vi "TDMS_Slicer.vi"() -> ()   [LabVIEW 2016]
doc: "TDMS로 저장된 파일을 읽고 추출함"
uses:
  Control/control_state.ctl
  <vilib>/Utility/error.llb/DialogType.ctl
panel:
  in  "Tach CH":i32=1
  out "RPM":dbl
  in  "Set input":i32
  in  "CH input":i32
  out "Measured time":string
  out "Error Out":errorcluster caption="에러 출력"
  in  "Error In":errorcluster caption="에러 입력"
  out "Channel number":string
  in  "Provious Set":bool
  in  "Next Set":bool
  in  "Provious CH":bool
  out "Data set number":string
  in  "Save name":string="FileNAME"
  out "TDMS Path":path
  out "Graph":waveform(dbl)(graph)
  out "TDMS_info":T1
  in  "END":bool
  in  "SAVE":bool
  in  "Next CH":bool
  in  "OPEN":bool
  # "TDMS read and extraction program by Kyuman Kim"
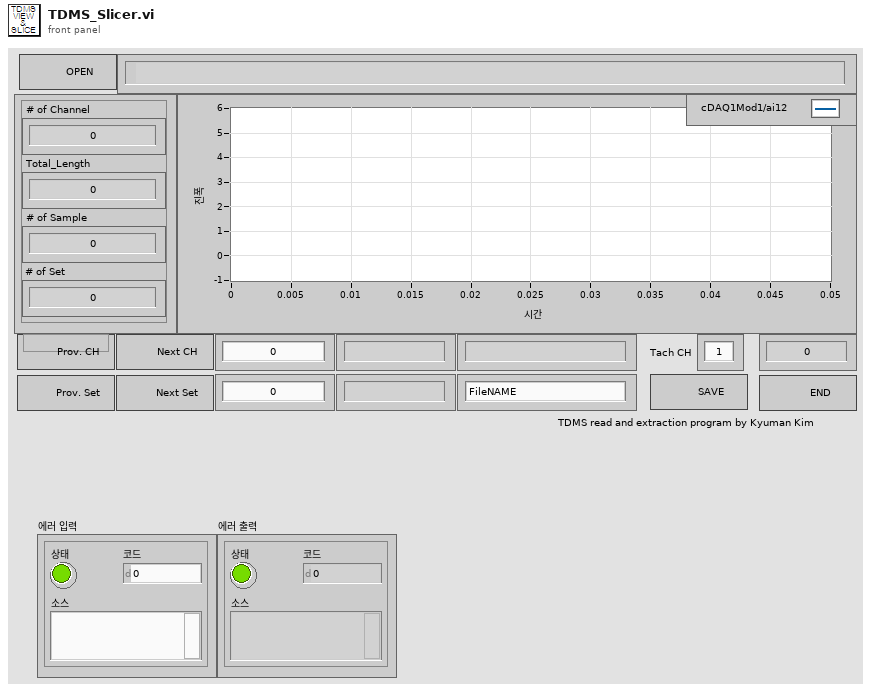
[diagram p1: front panel]
types:
  T1 = cluster{"# of Channel":i32, "Total_Length":u64, "# of Sample":i32, "# of Set":i32}
  T2 = typedef "control_state.ctl" = enum16{"Init", "Wait", "Setup", "Open", "Read", "Save", "End", "Error"}
  T3 = cluster{"# of Channel":i32, "Total_Length":u64, "# of Sample":i32, "# of Set":dbl}
  T4 = typedef "DialogType.ctl" = u16
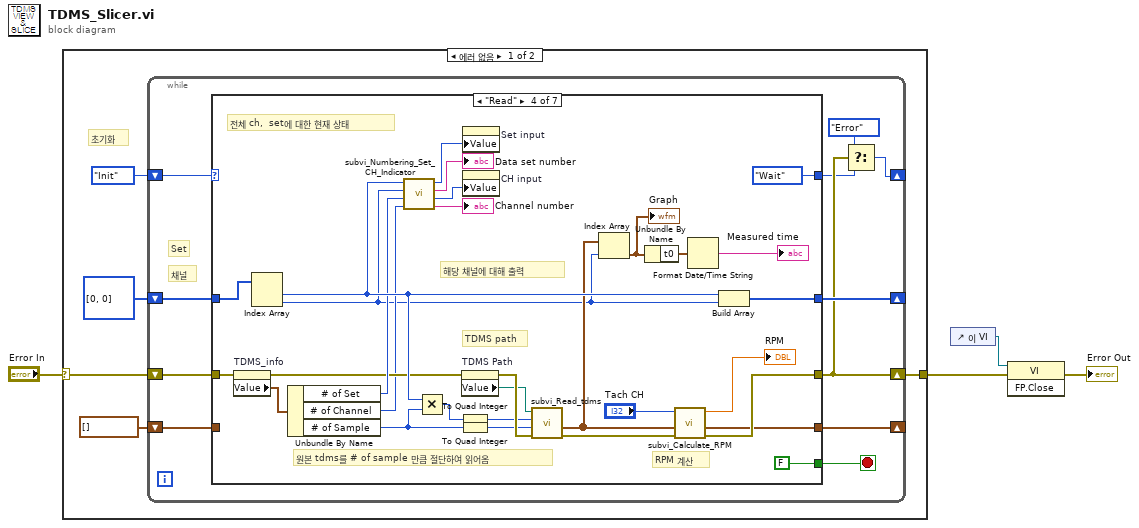
[diagram p0: block diagram]
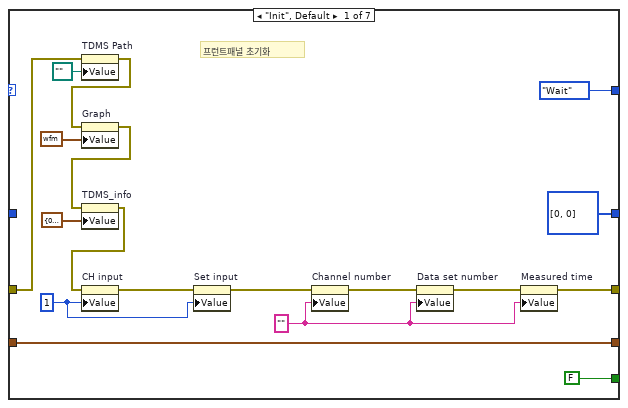
[diagram p2: hidden frame]
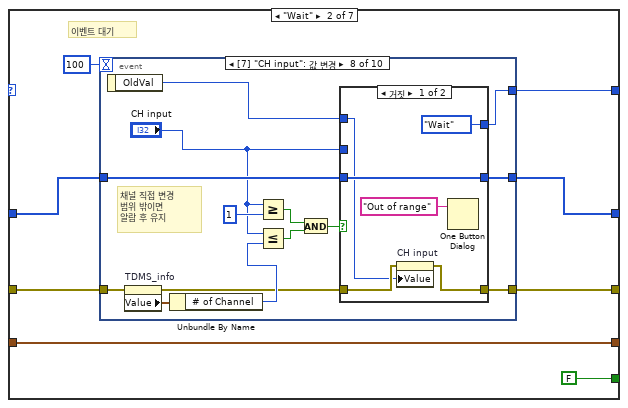
[diagram p3: hidden frame]
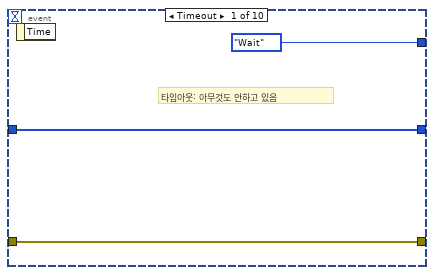
[diagram p4: hidden frame]
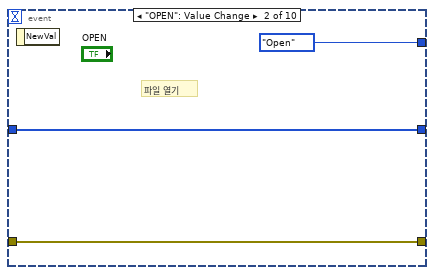
[diagram p5: hidden frame]
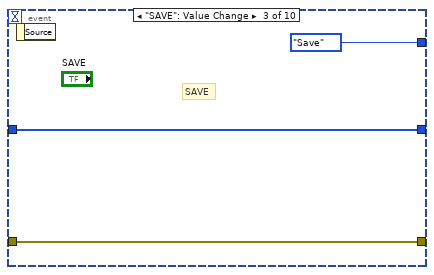
[diagram p6: hidden frame]
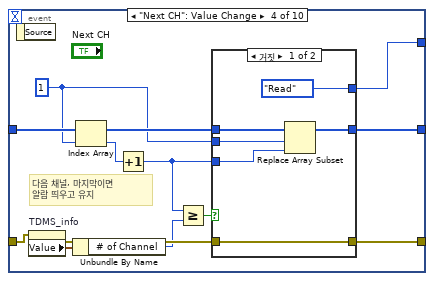
[diagram p7: hidden frame]
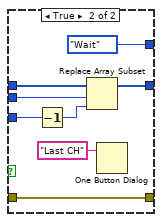
[diagram p8: hidden frame]
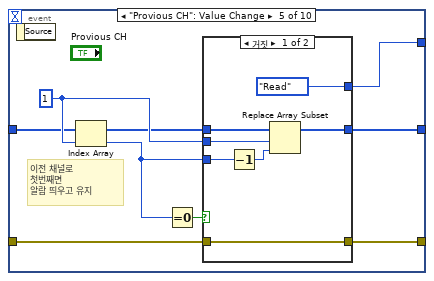
[diagram p9: hidden frame]
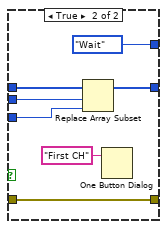
[diagram p10: hidden frame]
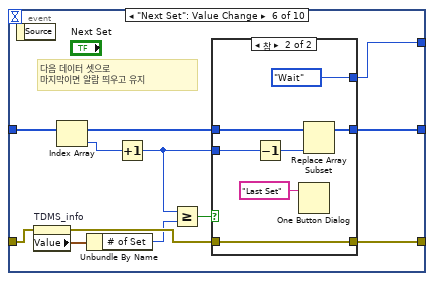
[diagram p11: hidden frame]
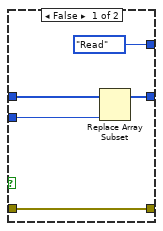
[diagram p12: hidden frame]
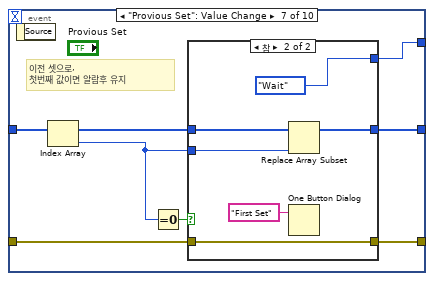
[diagram p13: hidden frame]
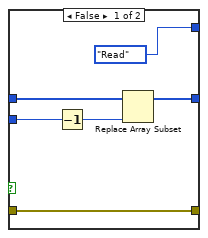
[diagram p14: hidden frame]
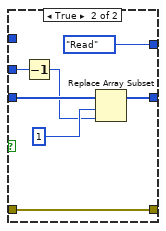
[diagram p15: hidden frame]
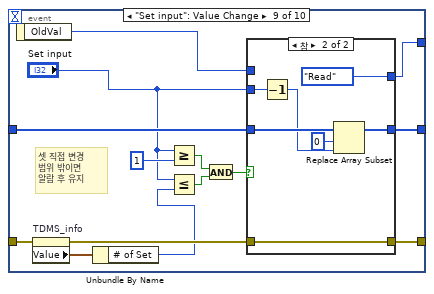
[diagram p16: hidden frame]
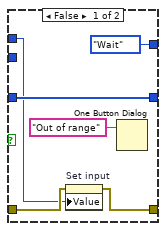
[diagram p17: hidden frame]
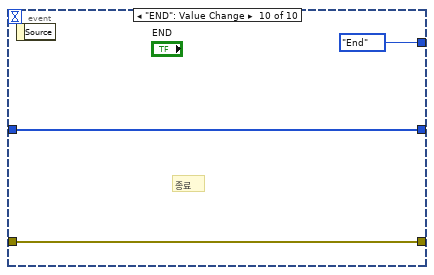
[diagram p18: hidden frame]
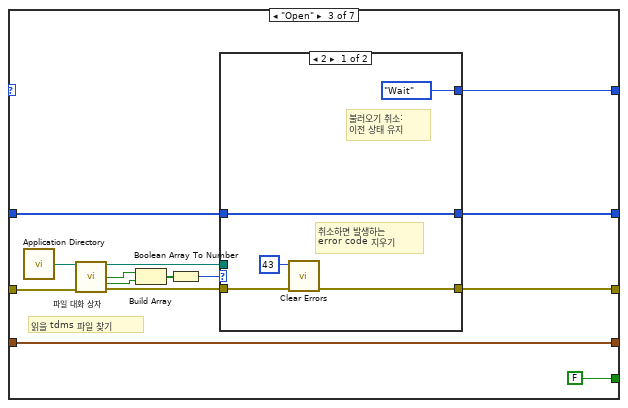
[diagram p19: hidden frame]
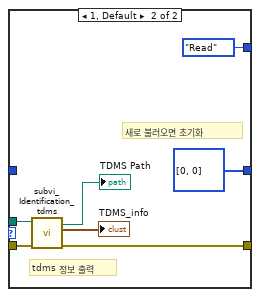
[diagram p20: hidden frame]
diagram:
  n1 = case shown="에러 없음" "Error In" {
    selector: "Error In" -> [w6 w309]
    tunnel: [w5 w309] -> w2
    frame No Error {
      # "초기화"
      n2 = while {
        shift-right: [w18] -> _
        shift-left: waveform(dbl)[] [] ("data") -> [w17]
        shift-right: [w16] -> _
        shift-left: i32[] [0, 0] -> [w19]
        shift-right: [w12] -> _
        shift-left: control_state."Init" ("열거형") -> [w20]
        shift-right: [w11] -> w5
        shift-left: w6 -> [w15]
        stop <- w14 stop-if-true
        # "채널"
        # "Set"
        n3 = case shown="\"Read\"" w20 {
          tunnel: w19 -> [_ w41 w205 w250 w265 _ _]
          tunnel: [FALSE FALSE FALSE FALSE FALSE w271 TRUE] -> w14
          tunnel: [w33 w43 w212 w231 w262 w277 waveform(dbl)[] [] ("data")] -> w18
          tunnel: w17 -> [w33 w43 w212 _ w262 w277 _]
          tunnel: [i32[] [0, 0] w42 w206 w248 w265 i32[] [] i32[] []] -> w16
          tunnel: [control_state."Wait" ("열거형") w44 w203 control_state."Wait" ("열거형") control_state."Wait" ("열거형") w274 control_state."Init" ("열거형")] -> w10
          tunnel: w15 -> [w38 w39 w211 w245 w267 w273 w303]
          tunnel: [w29 w40 w204 w234 w258 w272 w301] -> w11
          frame "Init", Default {
            w22 = 1 ("CH input")
            w23 = "" ("Channel number")
            # "프런트패널 초기화"
            n4 = property on="TDMS Path" class="Path"(error in=w38, "Value"=path "" ("TDMS Path")) -> (error out=w25:errorcluster)  [unwired: 1 in, 1 out]
            n5 = property on="Graph" class="WFGraph (엄격한)"(error in=w25, "Value"=waveform(dbl) {"t0"=timestamp(3735946803.3210297 s since 1904-01-01), "dt"=4.8824999999999954e-05, "Y"=[], "attributes"=variant("NI_ChannelName"=variant(string "cDAQ1Mod1/ai12"), "NI_UnitDescription"=variant(string "Volts"))} ("Graph")) -> (error out=w37:errorcluster)  [unwired: 1 in, 1 out]
            n6 = property on="TDMS_info" class="Clust (엄격한)"(error in=w37, "Value"=T3 {"# of Channel"=0, "Total_Length"=0, "# of Sample"=0, "# of Set"=0.0} ("TDMS_info")) -> (error out=w36:errorcluster)  [unwired: 1 in, 1 out]
            n7 = property on="CH input" class="DigNum (엄격한)"(error in=w36, "Value"=w22) -> (error out=w27:errorcluster)  [unwired: 1 in, 1 out]
            n8 = property on="Set input" class="DigNum (엄격한)"(error in=w27, "Value"=w22) -> (error out=w26:errorcluster)  [unwired: 1 in, 1 out]
            n9 = property on="Channel number" class="Str"(error in=w26, "Value"=w23) -> (error out=w30:errorcluster)  [unwired: 1 in, 1 out]
            n10 = property on="Data set number" class="Str"(error in=w30, "Value"=w23) -> (error out=w28:errorcluster)  [unwired: 1 in, 1 out]
            n11 = property on="Measured time" class="Str"(error in=w28, "Value"=w23) -> (error out=w29:errorcluster)  [unwired: 1 in, 1 out]
          }
          frame "Wait" {
            # "이벤트 대기"
            n12 = event shown="[7] \"CH input\": 값 변경" {
              selector: _ -> [_ _ _ _ _ _ _ _ _ _]
              dyn-events: _ -> [_ _ _ _ _ _ _ _ _ _]
              timeout: 100 -> [_ _ _ _ _ _ _ _ _ _]
              tunnel: [control_state."Wait" ("열거형") control_state."Open" ("열거형") control_state."Save" ("열거형") w62 w85 w106 w130 w159 w175 control_state."End" ("열거형")] -> w44
              tunnel: w41 -> [w48 w51 w54 w66 w88 w112 w133 w158 w178 w201]
              tunnel: [w48 w51 w54 w63 w87 w111 w132 w157 w176 w201] -> w42
              tunnel: [w47 w50 w53 w56 w82 w104 w128 w153 w183 w200] -> w40
              tunnel: w39 -> [w47 w50 w53 w57 w83 w105 w127 w154 w182 w200]
              event Timeout {
                # "타임아웃: 아무것도 안하고 있음"
                n13 = event-data() -> ()  [unwired: 1 in, 1 out]
              }
              event "OPEN": Value Change {
                # "파일 열기"
                n14 = event-data() -> ()  [unwired: 1 in, 1 out]
              }
              event "SAVE": Value Change {
                # "SAVE"
                n15 = event-data() -> ()  [unwired: 1 in, 1 out]
              }
              event "Next CH": Value Change {
                w64 = 1 ("인덱스")
                # "다음 채널, 마지막이면\n알람 띄우고 유지"
                n16 = event-data() -> ()  [unwired: 1 in, 1 out]
                n17 = property on="TDMS_info" class="Clust (엄격한)"(error in=w57) -> (error out=w67:errorcluster, "Value"=w61:T1)  [unwired: 1 in, 1 out]
                n18 = Unbundle By Name(w61) -> ("# of Channel"=w60:i32)
                n19 = Index Array(array=w66, index=w64) -> (element=w65:i32)
                n20 = Increment(x=w65) -> (x+1=w58:i32)
                n21 = Greater Or Equal?(x=w58, y=w60) -> (x >= y?=w59:bool)
                n22 = case shown="거짓" w59 {
                  tunnel: w66 -> [w72 w81]
                  tunnel: w58 -> [w70 w80]
                  tunnel: w64 -> [w71 w79]
                  tunnel: [w73 w78] -> w63
                  tunnel: [control_state."Read" ("열거형") control_state."Wait" ("열거형")] -> w62
                  tunnel: w67 -> [w68 w74]
                  tunnel: [w68 w74] -> w56
                  frame False {
                    n23 = Replace Array Subset(array=w72, new element=w70, index=w71) -> (w73:i32[])
                  }
                  frame True {
                    n24 = Decrement(x=w80) -> (x-1=w76:i32)
                    n25 = Replace Array Subset(array=w81, new element=w76, index=w79) -> (w78:i32[])
                    n26 = One Button Dialog(message="Last CH" ("메시지")) -> ()  [unwired: 1 in, 1 out]
                  }
                }
              }
              event "Provious CH": Value Change {
                w89 = 1 ("인덱스")
                # "이전 채널로\n첫번째면\n알람 띄우고 유지"
                n27 = event-data() -> ()  [unwired: 1 in, 1 out]
                n28 = Index Array(array=w88, index=w89) -> (element=w84:i32)
                n29 = Equal To 0?(x=w84) -> (x = 0?=w86:bool)
                n30 = case shown="거짓" w86 {
                  tunnel: w84 -> [w95 w98]
                  tunnel: w89 -> [w96 w103]
                  tunnel: w88 -> [w93 w102]
                  tunnel: [w94 w101] -> w87
                  tunnel: [control_state."Read" ("열거형") control_state."Wait" ("열거형")] -> w85
                  tunnel: w83 -> [w90 w97]
                  tunnel: [w90 w97] -> w82
                  frame False {
                    n31 = Decrement(x=w95) -> (x-1=w91:i32)
                    n32 = Replace Array Subset(array=w93, new element=w91, index=w96) -> (w94:i32[])
                  }
                  frame True {
                    n33 = Replace Array Subset(array=w102, new element=w98, index=w103) -> (w101:i32[])
                    n34 = One Button Dialog(message="First CH" ("메시지")) -> ()  [unwired: 1 in, 1 out]
                  }
                }
              }
              event "Next Set": Value Change {
                # "다음 데이터 셋으로\n마지막이면 알람 띄우고 유지"
                n35 = event-data() -> ()  [unwired: 1 in, 1 out]
                n36 = property on="TDMS_info" class="Clust (엄격한)"(error in=w105) -> (error out=w114:errorcluster, "Value"=w110:T1)  [unwired: 1 in, 1 out]
                n37 = Index Array(array=w112) -> (element=w113:i32)  [unwired: 1 in]
                n38 = Unbundle By Name(w110) -> ("# of Set"=w108:i32)
                n39 = Increment(x=w113) -> (x+1=w107:i32)
                n40 = Greater Or Equal?(x=w107, y=w108) -> (x >= y?=w109:bool)
                n41 = case shown="참" w109 {
                  tunnel: w107 -> [w117 w126]
                  tunnel: w112 -> [w119 w125]
                  tunnel: [w118 w124] -> w111
                  tunnel: [control_state."Read" ("열거형") control_state."Wait" ("열거형")] -> w106
                  tunnel: [w115 w120] -> w104
                  tunnel: w114 -> [w115 w120]
                  frame False {
                    n42 = Replace Array Subset(array=w119, new element=w117) -> (w118:i32[])  [unwired: 1 in]
                  }
                  frame True {
                    n43 = Decrement(x=w126) -> (x-1=w123:i32)
                    n44 = One Button Dialog(message="Last Set" ("메시지")) -> ()  [unwired: 1 in, 1 out]
                    n45 = Replace Array Subset(array=w125, new element=w123) -> (w124:i32[])  [unwired: 1 in]
                  }
                }
              }
              event "Provious Set": Value Change {
                # "이전 셋으로,\n첫번째 값이면 알람후 유지"
                n46 = event-data() -> ()  [unwired: 1 in, 1 out]
                n47 = Index Array(array=w133) -> (element=w129:i32)  [unwired: 1 in]
                n48 = Equal To 0?(x=w129) -> (x = 0?=w131:bool)
                n49 = case shown="참" w131 {
                  tunnel: w133 -> [w138 w145]
                  tunnel: [w137 w144] -> w132
                  tunnel: w129 -> [w139 w141]
                  tunnel: [control_state."Read" ("열거형") control_state."Wait" ("열거형")] -> w130
                  tunnel: [w134 w140] -> w128
                  tunnel: w127 -> [w134 w140]
                  frame False {
                    n50 = Decrement(x=w139) -> (x-1=w135:i32)
                    n51 = Replace Array Subset(array=w138, new element=w135) -> (w137:i32[])  [unwired: 1 in]
                  }
                  frame True {
                    n52 = Replace Array Subset(array=w145, new element=w141) -> (w144:i32[])  [unwired: 1 in]
                    n53 = One Button Dialog(message="First Set" ("메시지")) -> ()  [unwired: 1 in, 1 out]
                  }
                }
              }
              event "CH input": Value Change {
                # "채널 직접 변경\n범위 밖이면\n알람 후 유지"
                n54 = event-data() -> ("OldVal"=w148:i32)  [unwired: 1 in]
                n55 = property on="TDMS_info" class="Clust (엄격한)"(error in=w154) -> (error out=w147:errorcluster, "Value"=w156:T1)  [unwired: 1 in, 1 out]
                n56 = Unbundle By Name(w156) -> ("# of Channel"=w149:i32)
                n57 = Greater Or Equal?(x="CH input", y=1) -> (x >= y?=w151:bool)
                n58 = Less Or Equal?(x="CH input", y=w149) -> (x <= y?=w150:bool)
                n59 = And(x=w151, y=w150) -> (x .and. y?=w152:bool)
                n60 = case shown="거짓" w152 {
                  tunnel: [control_state."Wait" ("열거형") control_state."Read" ("열거형")] -> w159
                  tunnel: w158 -> [w164 w171]
                  tunnel: [w164 w170] -> w157
                  tunnel: w147 -> [w162 w167]
                  tunnel: [w161 w167] -> w153
                  tunnel: "CH input" -> [_ w166]
                  tunnel: w148 -> [w160 _]
                  frame False {
                    n61 = property on="CH input" class="DigNum (엄격한)"(error in=w162, "Value"=w160) -> (error out=w161:errorcluster)  [unwired: 1 in, 1 out]
                    n62 = One Button Dialog(message="Out of range" ("메시지")) -> ()  [unwired: 1 in, 1 out]
                  }
                  frame True {
                    n63 = Decrement(x=w166) -> (x-1=w168:i32)
                    n64 = Replace Array Subset(array=w171, new element=w168, index=1 ("인덱스")) -> (w170:i32[])
                  }
                }
              }
              event "Set input": Value Change {
                # "셋 직접 변경\n범위 밖이면\n알람 후 유지"
                n65 = event-data() -> ("OldVal"=w177:i32)  [unwired: 1 in]
                n66 = property on="TDMS_info" class="Clust (엄격한)"(error in=w182) -> (error out=w181:errorcluster, "Value"=w180:T1)  [unwired: 1 in, 1 out]
                n67 = Unbundle By Name(w180) -> ("# of Set"=w179:i32)
                n68 = Greater Or Equal?(x="Set input", y=1) -> (x >= y?=w185:bool)
                n69 = Less Or Equal?(x="Set input", y=w179) -> (x <= y?=w184:bool)
                n70 = And(x=w185, y=w184) -> (x .and. y?=w174:bool)
                n71 = case shown="참" w174 {
                  tunnel: [control_state."Wait" ("열거형") control_state."Read" ("열거형")] -> w175
                  tunnel: w178 -> [w191 w198]
                  tunnel: [w191 w197] -> w176
                  tunnel: w181 -> [w189 w194]
                  tunnel: [w188 w194] -> w183
                  tunnel: w177 -> [w187 _]
                  tunnel: "Set input" -> [_ w193]
                  frame False {
                    n72 = property on="Set input" class="DigNum (엄격한)"(error in=w189, "Value"=w187) -> (error out=w188:errorcluster)  [unwired: 1 in, 1 out]
                    n73 = One Button Dialog(message="Out of range" ("메시지")) -> ()  [unwired: 1 in, 1 out]
                  }
                  frame True {
                    n74 = Decrement(x=w193) -> (x-1=w195:i32)
                    n75 = Replace Array Subset(array=w198, new element=w195, index=0 ("인덱스")) -> (w197:i32[])
                  }
                }
              }
              event "END": Value Change {
                # "종료"
                n76 = event-data() -> ()  [unwired: 1 in, 1 out]
              }
            }
          }
          frame "Open" {
            # "읽을 tdms 파일 찾기"
            n77 = call <vilib>:"Application Directory.vi"() -> ("Application Directory"=w216:path)
            n78 = call "파일 대화 상자"("start path"=w216, "error in"=w211) -> ("selected path"=w215:path, "exists"=w210:bool, "cancelled"=w209:bool, "error out"=w214:errorcluster)  [unwired: 10 in]
            n79 = Build Array(w210, w209) -> (w208:bool[])
            n80 = Boolean Array To Number(Boolean array=w208) -> (number=w207:u32)
            n81 = case shown="2" w207 {
              tunnel: w215 -> [_ w228]
              tunnel: w214 -> [w219 w227]
              tunnel: [control_state."Wait" ("열거형") control_state."Read" ("열거형")] -> w203
              tunnel: [w218 w225] -> w204
              tunnel: [w220 i32[] [0, 0]] -> w206
              tunnel: w205 -> [w220 _]
              frame 2 {
                # "취소하면 발생하는 \nerror code 지우기"
                # "불러오기 취소:\n이전 상태 유지"
                n82 = call <vilib>:"Clear Errors.vi"("error in (no error)"=w219, "specific error code to clear (0: all)"=43) -> ("error out"=w218:errorcluster)  [unwired: 4 in, 1 out]
              }
              frame 1, Default {
                # "새로 불러오면 초기화"
                # "tdms 정보 출력"
                n83 = call "subvi_Identification_tdms.vi"("Error In"=w227, "Path in"=w228) -> ("Error Out"=w225:errorcluster, "TDMS_info"=→"TDMS_info":T1, "Path out"=→"TDMS Path":path)  [unwired: 7 in]
              }
            }
          }
          frame "Read" {
            # "RPM 계산"
            # "TDMS path"
            # "해당 채널에 대해 출력"
            # "원본 tdms를 # of sample 만큼 절단하여 읽어옴"
            # "전체 ch,  set에 대한 현재 상태"
            n84 = property on="TDMS_info" class="Clust (엄격한)"(error in=w245) -> (error out=w240:errorcluster, "Value"=w256:T1)  [unwired: 1 in, 1 out]
            n85 = Index Array(array=w250) -> (element #1=w249:i32, element #2=w229:i32)  [unwired: 2 in]
            n86 = Unbundle By Name(w256) -> ("# of Set"=w241:i32, "# of Channel"=w235:i32, "# of Sample"=w253:i32)
            n87 = call "subvi_Numbering_Set_CH_Indicator.vi"("# of Channel"=w235, "# of Set"=w241, "CH data"=w229, "Set data"=w249) -> ("CH state"=→"Channel number":string, "CH value"=w237:i32, "Set state"=→"Data set number":string, "Set value"=w238:i32)  [unwired: 4 in]
            n88 = Multiply(x=w249, y=w253) -> (x*y=w252:i32)
            n89 = To Quad Integer(1:w252) -> (0:w254:i64)
            n90 = To Quad Integer(1:w253) -> (0:w255:i64)
            n91 = property on="TDMS Path" class="Path"(error in=w240) -> (error out=w257:errorcluster, "Value"=w239:path)  [unwired: 1 in, 1 out]
            n92 = property on="Set input" class="DigNum (엄격한)"("Value"=w238) -> ()  [unwired: 2 in, 2 out]
            n93 = property on="CH input" class="DigNum (엄격한)"("Value"=w237) -> ()  [unwired: 2 in, 2 out]
            n94 = call "subvi_Read_tdms.vi"("Error In"=w257, "카운트(-1: 전체)"=w255, "오프셋(0)"=w254, "selected path"=w239) -> ("Error Out"=w233:errorcluster, "data"=w231:waveform(dbl)[])  [unwired: 6 in]
            n95 = Index Array(array=w231, index=w229) -> (element=w244:waveform(dbl))
            "Graph" <- w244
            n96 = Unbundle By Name(w244) -> ("t0"=w243:timestamp)
            n97 = call "subvi_Calculate_RPM.vi"("에러 입력"=w233, "data"=w231, "Tach CH"="Tach CH") -> ("에러 출력"=w234:errorcluster, "RPM"=→"RPM":dbl)  [unwired: 7 in]
            n98 = Format Date/Time String(seconds (now)=w243) -> (date/time string=→"Measured time":string)  [unwired: 2 in]
            n99 = Build Array(w249, w229) -> (w248:i32[])
          }
          frame "Save" {
            # "어플리케이션 경로"
            # "그룹이름"
            # "어플리케이션 경로 밑에 TDMS_Sliced 폴더에 날짜_이름으로 저장"
            n100 = call <vilib>:"Application Directory.vi"() -> ("Application Directory"=w260:path)
            n101 = call "subvi_Save_tdms.vi"("data"=w262, "그룹 이름"="Sliced data" ("그룹 이름 입력(제목없음)"), "Error In"=w267, "Save name"="Save name", "appended path"=w260) -> ("Error Out"=w259:errorcluster)  [unwired: 6 in]
            n102 = flat-sequence {
              tunnel: [w268] -> w258
              tunnel: w259 -> [w268]
              frame #0 {
                n103 = One Button Dialog(message="Sliced TDMS\nSAVED" ("메시지")) -> ()  [unwired: 1 in, 1 out]
              }
            }
          }
          frame "End" {
            n104 = Two Button Dialog(message="끝냅니다" ("메시지")) -> (T button?=w275:bool)  [unwired: 2 in]
            n105 = case shown="거짓" w275 {
              tunnel: w273 -> [w280 w285]
              tunnel: [control_state."Wait" ("열거형") control_state."Init" ("열거형")] -> w274
              tunnel: [w280 w289] -> w272
              tunnel: [FALSE TRUE] -> w271
              frame False {
                # "아무것도 하지 않고 wait 이동"
              }
              frame True {
                w283 = "" ("Channel number")
                # "종료 전 초기화"
                n106 = property on="TDMS Path" class="Path"(error in=w285, "Value"=path "" ("TDMS Path")) -> (error out=w284:errorcluster)  [unwired: 1 in, 1 out]
                n107 = property on="Graph" class="WFGraph (엄격한)"(error in=w284, "Value"=waveform(dbl) {"t0"=timestamp(3735946803.3210297 s since 1904-01-01), "dt"=4.8824999999999954e-05, "Y"=[], "attributes"=variant("NI_ChannelName"=variant(string "cDAQ1Mod1/ai12"), "NI_UnitDescription"=variant(string "Volts"))} ("Graph")) -> (error out=w293:errorcluster)  [unwired: 1 in, 1 out]
                n108 = property on="TDMS_info" class="Clust (엄격한)"(error in=w293, "Value"=T3 {"# of Channel"=0, "Total_Length"=0, "# of Sample"=0, "# of Set"=0.0} ("TDMS_info")) -> (error out=w292:errorcluster)  [unwired: 1 in, 1 out]
                n109 = property on="CH input" class="DigNum (엄격한)"(error in=w292, "Value"=1 ("CH input")) -> (error out=w288:errorcluster)  [unwired: 1 in, 1 out]
                n110 = property on="Set input" class="DigNum (엄격한)"(error in=w288, "Value"=1 ("Set input")) -> (error out=w287:errorcluster)  [unwired: 1 in, 1 out]
                n111 = property on="Channel number" class="Str"(error in=w287, "Value"=w283) -> (error out=w291:errorcluster)  [unwired: 1 in, 1 out]
                n112 = property on="Data set number" class="Str"(error in=w291, "Value"=w283) -> (error out=w290:errorcluster)  [unwired: 1 in, 1 out]
                n113 = property on="Measured time" class="Str"(error in=w290, "Value"=w283) -> (error out=w289:errorcluster)  [unwired: 1 in, 1 out]
              }
            }
          }
          frame "Error" {
            w304 = T4 3 items=["대화 상자 없음", "확인 메시지", "메시지 지속 또는 정지", "확인 메시지 + 경고", "지속/정지 + 경고"] ("type of dialog (OK msg:1)")
            n114 = call <vilib>:"General Error Handler.vi"("type of dialog (OK msg:1)"=w304, "error in (no error)"=w303) -> ("error out"=w300:errorcluster)  [unwired: 9 in, 4 out]
            n115 = flat-sequence {
              tunnel: w300 -> [w308]
              tunnel: [w308] -> w298
              frame #0 {
                n116 = One Button Dialog(message="에러로 인해서 \n종료합니다." ("메시지")) -> ()  [unwired: 1 in, 1 out]
              }
            }
            n117 = call <vilib>:"Clear Errors.vi"("error in (no error)"=w298) -> ("error out"=w301:errorcluster)  [unwired: 5 in, 1 out]
          }
        }
        n118 = Select(t=control_state."Error" ("열거형"), s=w11, f=w10) -> (s? t:f=w12:T2)
      }
    }
    frame Error {
    }
  }
  n119 = control-ref of="이 VI"() -> (w1:refnum<vi>)
  n120 = invoke class="VI" method="FP.Close"(reference=w1, error in=w2) -> (error out=→"Error Out":errorcluster)  [unwired: 1 in, 2 out]
